vi "ExampleVI_VISImage.vi"() -> ()   [LabVIEW 2013]
uses:
  <vilib>/picture/picture.llb/imagedata.ctl
panel:
  out "Width":i32=2048
  out "Height":i32=1536
  in  "GETIMAGE - Button":bool
  in  "EXIT - Button":bool
  in  "Menüring":u32(ring) items=["t885-1(2078204)"=2078204]
  out "Boolesch":bool
  in  "CONNECT - BUTTON":bool
  out "new picture 3":picture
  out "Fehler (Ausgang)":errorcluster caption="ErrorOut"
  # "CONNECTION"
  # "VIS IMAGE"
  # "Height"
  # "Width"
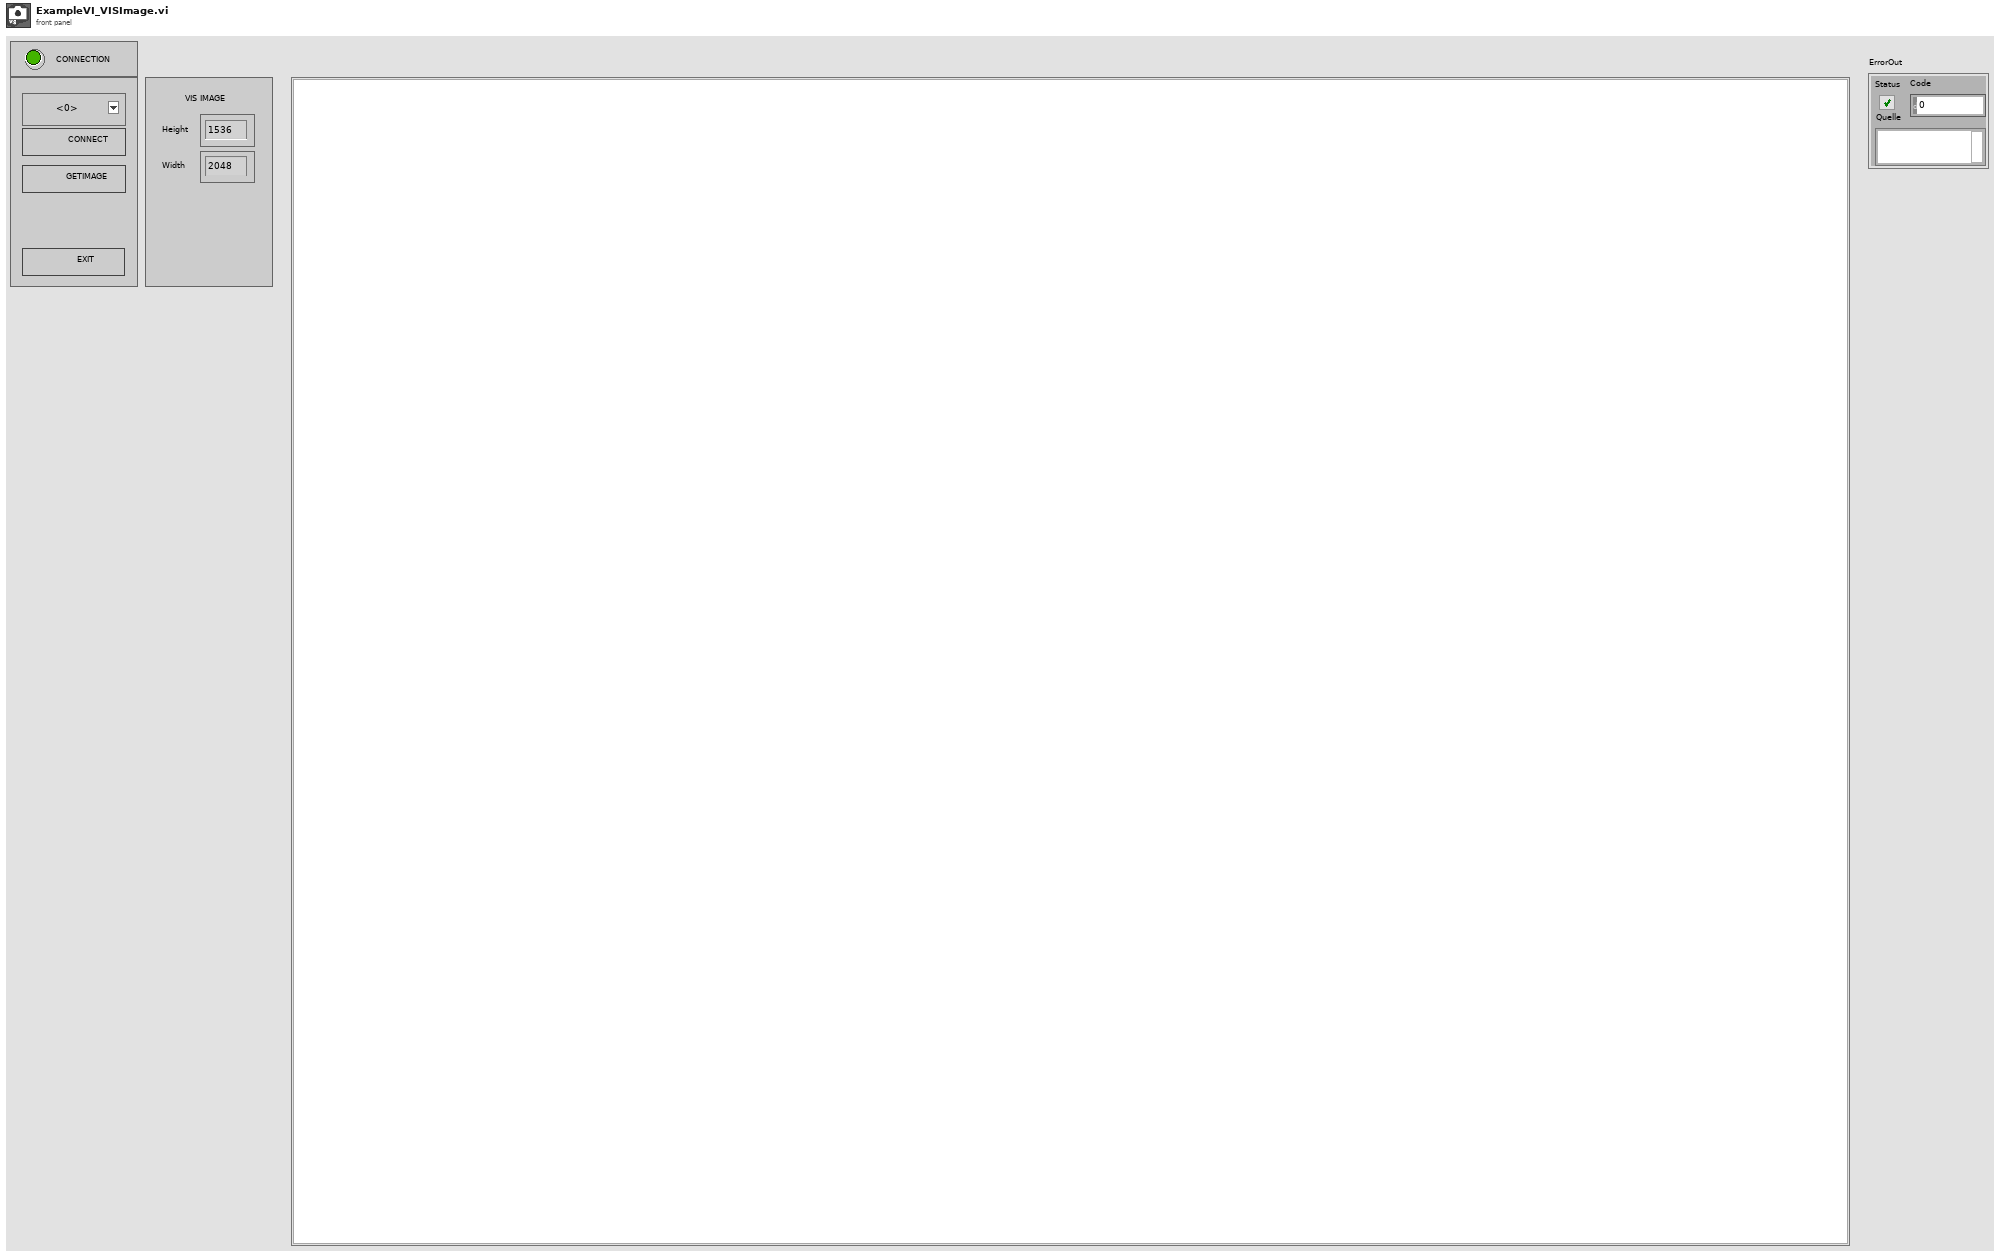
[diagram p1: front panel]
types:
  T1 = typedef "imagedata.ctl" = cluster{"image type":i32, "image depth":i32, "image":u8[], "mask":u8[], "colors":u32[], "Rectangle":cluster{"left":i16, "top":i16, "right":i16, "bottom":i16}}
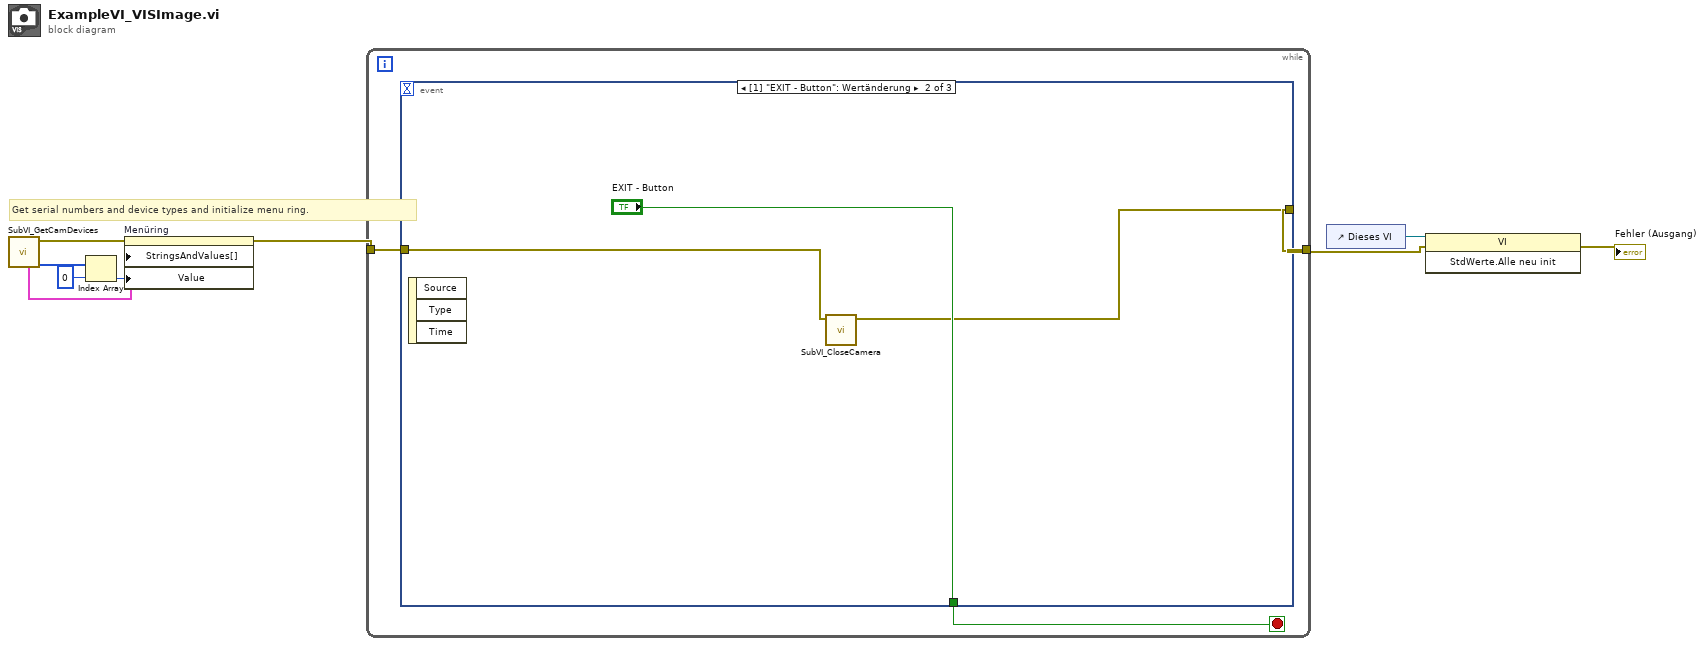
[diagram p0: block diagram]
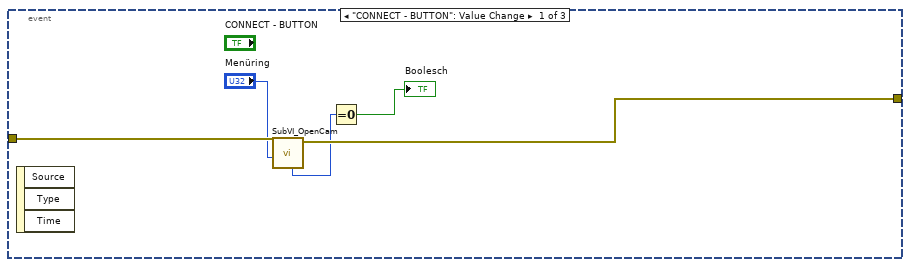
[diagram p2: hidden frame]
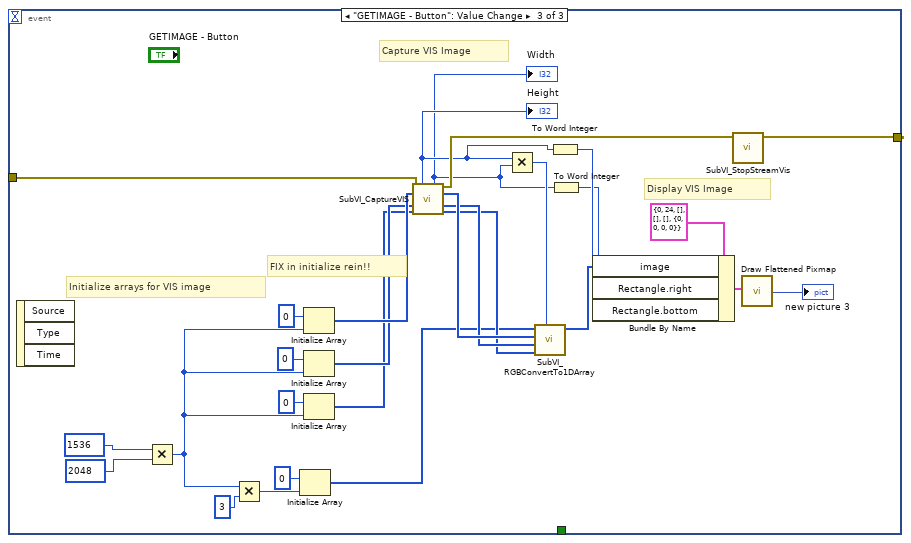
[diagram p3: hidden frame]
diagram:
  # "Get serial numbers and device types and initialize menu ring."
  n1 = call "SubVI_GetCamDevices.vi"() -> ("au32CameraSerials"=w6:u32[], "ErrorOut"=w8:errorcluster, "strCameraDeviceType"=w4:cluster{string, "Output":u32}[])  [unwired: 7 in, 2 out]
  n2 = Index Array(array=w6, index=0 ("Index")) -> (element=w5:u32)
  n3 = property on="Menüring" class="Ring (strikt)"(error in=w8, "StringsAndValues[]"=w4, "Value"=w5) -> (error out=w9:errorcluster)  [unwired: 1 in, 1 out]
  n4 = while {
    tunnel: w9 -> [w12]
    tunnel: [w10] -> w2
    stop <- w11 stop-if-true
    n5 = event shown="[1] \"EXIT - Button\": Wertänderung" {
      selector: _ -> [_ _ _]
      dyn-events: _ -> [_ _ _]
      timeout: _ -> [_ _ _]
      tunnel: w12 -> [w15 w19 w41]
      tunnel: [w16 w18 w25] -> w10
      tunnel: [_ "EXIT - Button" _] -> w11
      event "CONNECT - BUTTON": Value Change {
        n6 = event-data() -> ()  [unwired: 1 in, 3 out]
        n7 = call "SubVI_OpenCam.vi"("u32SerialNumber"="Menüring", "ErrorIn"=w15) -> ("ErrorOut"=w16:errorcluster, "u8Status"=w13:u8)  [unwired: 8 in]
        n8 = Equal To 0?(x=w13) -> (x = 0?=→"Boolesch":bool)
      }
      event "EXIT - Button": Value Change {
        n9 = event-data() -> ()  [unwired: 1 in, 3 out]
        n10 = call "SubVI_CloseCamera.vi"("ErrorIn"=w19) -> ("ErrorOut"=w18:errorcluster)  [unwired: 9 in, 1 out]
      }
      event "GETIMAGE - Button": Value Change {
        # "Initialize arrays for VIS image"
        # "FIX in initialize rein!!"
        # "Capture VIS Image"
        # "Display VIS Image"
        n11 = event-data() -> ()  [unwired: 1 in, 3 out]
        n12 = Multiply(x=1536 ("Height 2"), y=2048 ("Width 2")) -> (x*y=w28:i32)
        n13 = Multiply(x=w28, y=3) -> (x*y=w35:i32)
        n14 = Initialize Array(u8 0 ("Element"), w35) -> (w32:u8[])
        n15 = Initialize Array ("Array initialisieren")(u8 0 ("Element"), w28) -> (w31:u8[])
        n16 = Initialize Array(u8 0 ("Element"), w28) -> (w30:u8[])
        n17 = Initialize Array(u8 0 ("Element"), w28) -> (w29:u8[])
        n18 = call "SubVI_CaptureVIS.vi"("ErrorIn"=w41, "au8Channel-B"=w31, "au8Channel-G"=w30, "au8Channel-R"=w29) -> ("i32VisHeight"=w24:i32, "i32VisWidth"=w22:i32, "ErrorOut"=w26:errorcluster, "au8Channel-B"=w44:u8[], "au8Channel-G"=w43:u8[], "au8Channel-R"=w42:u8[])  [unwired: 5 in, 1 out]
        "Height" <- w24
        "Width" <- w22
        n19 = Multiply(x=w22, y=w24) -> (x*y=w27:i32)
        n20 = call "SubVI_RGBConvertTo1DArray.vi"("i32PixelAmount"=w27, "au8Channel-R"=w42, "au8Channel-G"=w43, "au8Channel-B"=w44, "au8SerializedImage[in]"=w32) -> ("au8SerializedImage[out]"=w45:u8[])  [unwired: 6 in]
        n21 = To Word Integer(number=w24) -> (16bit integer=w23:i16)
        n22 = To Word Integer(number=w22) -> (16bit integer=w21:i16)
        n23 = Bundle By Name(cluster=T1 {"image type"=0, "image depth"=24, "image"=[], "mask"=[], "colors"=[], "Rectangle"={"left"=0, "top"=0, "right"=0, "bottom"=0}} ("image data"), "image"=w45, "Rectangle.right"=w21, "Rectangle.bottom"=w23) -> (w47:T1)
        n24 = call "SubVI_StopStreamVis.vi"("ErrorIn"=w26) -> ("ErrorOut"=w25:errorcluster)  [unwired: 9 in, 1 out]
        n25 = call <vilib>:"Draw Flattened Pixmap.vi"("image data"=w47) -> ("new picture"=→"new picture 3":picture)  [unwired: 8 in]
      }
    }
  }
  n26 = control-ref of="Dieses VI"() -> (w3:refnum<vi>)
  n27 = invoke class="VI" method="StdWerte.Alle neu init"(reference=w3, error in=w2) -> (error out=→"Fehler (Ausgang)":errorcluster)  [unwired: 1 in, 2 out]
